vi "AMC Flush Message Queue.vi"(7 "error in (no error)":errorcluster, 10 "Message Queue in":T1) -> (0 "error out":errorcluster, 3 "Message Queue out":T1)   [LabVIEW 2011, in "ART2 Test Panel.lvlib" / "TLB_Dependencies.lvlib"]
uses:
  TLB_Dependencies.lvlib
  amc_Message Queue.ctl
  amc_Message.ctl
  Users/rkidagan/Dropbox/Atheros/ART2/Development/ART2 Test Panel/ART2 Test Panel/Components/Dependencies.llb/Keyed Array.ctl
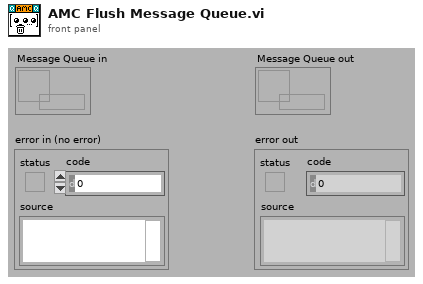
[diagram p1: front panel]
types:
  T1 = typedef "ART2 Test Panel.lvlib/TLB_Dependencies.lvlib/amc_Message Queue.ctl" = refnum<queue>
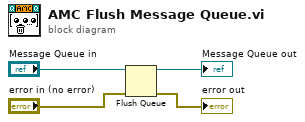
[diagram p0: block diagram]
diagram:
  n1 = Flush Queue(queue="Message Queue in", error in (no error)="error in (no error)") -> (queue out=→"Message Queue out":T1, error out=→"error out":errorcluster)  [unwired: 1 out]
